vi "Bilinear Interpolation.vi"(10 "a":dbl, 11 "Image Data In":T1) -> (3 "Image Data Out":T1)   [LabVIEW 2015]
uses:
  <vilib>/picture/picture.llb/imagedata.ctl
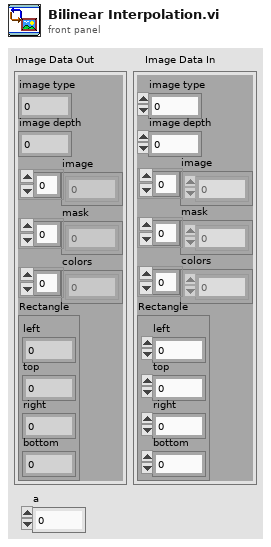
[diagram p1: front panel]
types:
  T1 = typedef "imagedata.ctl" = cluster{"image type":i32, "image depth":i32, "image":u8[], "mask":u8[], "colors":u32[], "Rectangle":cluster{"left":i16, "top":i16, "right":i16, "bottom":i16}}
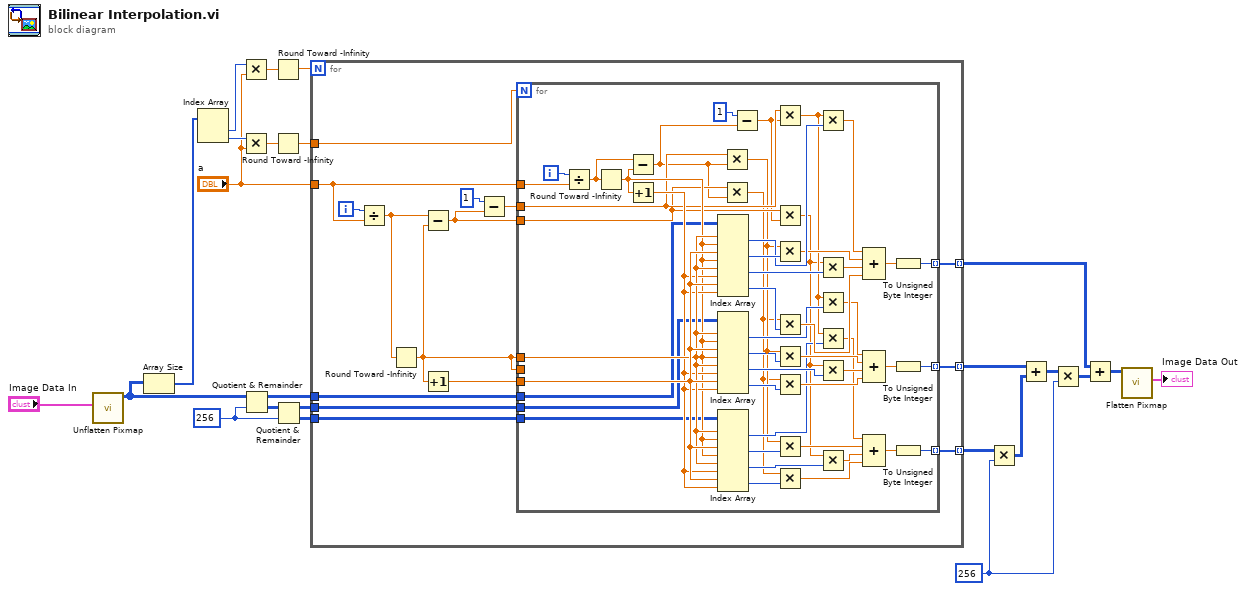
[diagram p0: block diagram]
diagram:
  w3 = 256
  w4 = 256
  n1 = call <vilib>:"Unflatten Pixmap.vi"("image data"="Image Data In") -> ("24-bit pixmap"=w5:u32[][])  [unwired: 4 in, 6 out]
  n2 = Array Size(array=w5) -> (size(s)=w24:i32[])
  n3 = Index Array(array=w24) -> (element #1=w23:i32, element #2=w22:i32)  [unwired: 2 in]
  n4 = Multiply(x=w23, y="a") -> (x*y=w21:dbl)
  n5 = Multiply(x=w22, y="a") -> (x*y=w20:dbl)
  n6 = Quotient & Remainder(x=w5, y=w4) -> (x-y*floor(x/y)=w15:u32[][], floor(x/y)=w16:u32[][])
  n7 = Round Toward -Infinity(1:w21) -> (0:w19:dbl)
  n8 = Round Toward -Infinity(1:w20) -> (0:w18:dbl)
  n9 = Quotient & Remainder(x=w16, y=w4) -> (x-y*floor(x/y)=w14:u32[][], floor(x/y)=w13:u32[][])
  n10 = for {
    N: w19 -> [_]
    tunnel: "a" -> [w37]
    tunnel: w18 -> [w38]
    tunnel: w15 -> [w29]
    tunnel: w14 -> [w30]
    tunnel: w13 -> [w31]
    tunnel: [w28] -> w8 mode=indexing
    tunnel: [w27] -> w10 mode=indexing
    tunnel: [w26] -> w12 mode=indexing
    i -> [w25]
    n11 = Divide(x=w25, y=w37) -> (x/y=w39:dbl)
    n12 = Round Toward -Infinity(1:w39) -> (0:w35:dbl)
    n13 = Subtract(x=w39, y=w35) -> (x-y=w33:dbl)
    n14 = Increment(x=w35) -> (x+1=w36:dbl)
    n15 = Subtract(x=1, y=w33) -> (x-y=w32:dbl)
    n16 = for {
      N: w38 -> [_]
      tunnel: w37 -> [w88]
      tunnel: w35 -> [_]
      tunnel: w36 -> [w85]
      tunnel: w35 -> [w84]
      tunnel: w30 -> [w81]
      tunnel: w33 -> [w78]
      tunnel: w32 -> [w79]
      tunnel: w31 -> [w75]
      tunnel: w29 -> [w74]
      tunnel: [w45] -> w28 mode=indexing
      tunnel: [w44] -> w27 mode=indexing
      tunnel: [w43] -> w26 mode=indexing
      i -> [w87]
      n17 = Divide(x=w87, y=w88) -> (x/y=w86:dbl)
      n18 = Round Toward -Infinity(1:w86) -> (0:w82:dbl)
      n19 = Subtract(x=w86, y=w82) -> (x-y=w76:dbl)
      n20 = Increment(x=w82) -> (x+1=w83:dbl)
      n21 = Index Array(array=w74, index (row) #1=w84, index (col) #1=w82, index (row) #2=w85, index (col) #2=w82, index (row) #3=w84, index (col) #3=w83, index (row) #4=w85, index (col) #4=w83) -> (element #1=w71:u32, element #2=w72:u32, element #3=w70:u32, element #4=w73:u32)
      n22 = Index Array(array=w81, index (row) #1=w84, index (col) #1=w82, index (row) #2=w85, index (col) #2=w82, index (row) #3=w84, index (col) #3=w83, index (row) #4=w85, index (col) #4=w83) -> (element #1=w58:u32, element #2=w59:u32, element #3=w60:u32, element #4=w61:u32)
      n23 = Index Array(array=w75, index (row) #1=w84, index (col) #1=w82, index (row) #2=w85, index (col) #2=w82, index (row) #3=w84, index (col) #3=w83, index (row) #4=w85, index (col) #4=w83) -> (element #1=w50:u32, element #2=w51:u32, element #3=w52:u32, element #4=w53:u32)
      n24 = Multiply(x=w79, y=w76) -> (x*y=w48:dbl)
      n25 = Multiply(x=w78, y=w76) -> (x*y=w46:dbl)
      n26 = Subtract(x=1, y=w76) -> (x-y=w77:dbl)
      n27 = Multiply(x=w79, y=w77) -> (x*y=w49:dbl)
      n28 = Multiply(x=w78, y=w77) -> (x*y=w47:dbl)
      n29 = Multiply(x=w48, y=w72) -> (x*y=w68:dbl)
      n30 = Multiply(x=w46, y=w73) -> (x*y=w66:dbl)
      n31 = Multiply(x=w48, y=w59) -> (x*y=w64:dbl)
      n32 = Multiply(x=w46, y=w61) -> (x*y=w62:dbl)
      n33 = Multiply(x=w48, y=w51) -> (x*y=w56:dbl)
      n34 = Multiply(x=w46, y=w53) -> (x*y=w54:dbl)
      n35 = Multiply(x=w49, y=w71) -> (x*y=w69:dbl)
      n36 = Multiply(x=w47, y=w70) -> (x*y=w67:dbl)
      n37 = Multiply(x=w49, y=w58) -> (x*y=w65:dbl)
      n38 = Multiply(x=w49, y=w50) -> (x*y=w57:dbl)
      n39 = Multiply(x=w47, y=w60) -> (x*y=w63:dbl)
      n40 = Multiply(x=w47, y=w52) -> (x*y=w55:dbl)
      n41 = Compound Arithmetic op=ADD(w69, w68, w67, w66) -> (w42:dbl)
      n42 = Compound Arithmetic op=ADD(w65, w64, w63, w62) -> (w41:dbl)
      n43 = Compound Arithmetic op=ADD(w57, w56, w55, w54) -> (w40:dbl)
      n44 = To Unsigned Byte Integer(number=w42) -> (unsigned 8bit integer=w45:u8)
      n45 = To Unsigned Byte Integer(number=w41) -> (unsigned 8bit integer=w44:u8)
      n46 = To Unsigned Byte Integer(number=w40) -> (unsigned 8bit integer=w43:u8)
    }
  }
  n47 = Multiply(x=w12, y=w3) -> (x*y=w11:i32[][])
  n48 = Add(x=w10, y=w11) -> (x+y=w9:i32[][])
  n49 = Multiply(x=w9, y=w3) -> (x*y=w7:i32[][])
  n50 = Add(x=w8, y=w7) -> (x+y=w6:i32[][])
  n51 = call <vilib>:"Flatten Pixmap.vi"("24-bit pixmap"=w6) -> ("image data"=→"Image Data Out":T1)  [unwired: 10 in]
